vi "Write MVIName.vi"(8 "error in (no error)":errorcluster, 10 "MVIName":string, 11 "MB Param in":refnum<class "Param.lvclass">) -> (0 "error out":errorcluster, 3 "MB Param out":refnum<class "Param.lvclass">)   [LabVIEW 2021, in "Param.lvlib" / "Param.lvclass"]
uses:
  Param.lvclass
  Param.lvclass/Param.ctl
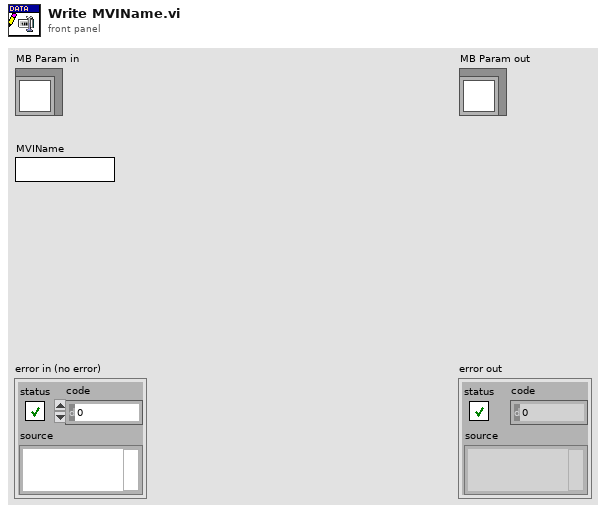
[diagram p1: front panel]
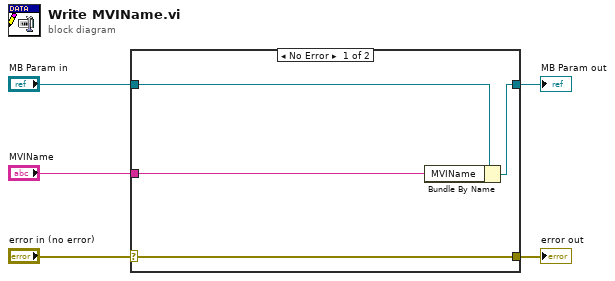
[diagram p0: block diagram]
diagram:
  n1 = case shown="No Error" "error in (no error)" {
    selector: "error in (no error)" -> [w9 w10]
    tunnel: [w9 w10] -> w4
    tunnel: [w7 w11] -> w2
    tunnel: "MB Param in" -> [w8 w11]
    tunnel: "MVIName" -> [w6 _]
    frame No Error {
      n2 = Bundle By Name(cluster=w8, "MVIName"=w6) -> (w7:refnum<class "Param.lvclass">)
    }
    frame Error {
    }
  }
  "error out" <- w4
  "MB Param out" <- w2
